vi "view_user_event.vi"(0 "State":string, 5 "Data":variant, 11 "error in (no error)":errorcluster, 13 "Operation":T1) -> (4 "Event Ref":refnum<user-event>, 15 "error out":errorcluster)   [LabVIEW 2020, in "simple_html_chat_ui.lvclass"]
uses:
  simple_html_chat_ui.lvclass
  ui_user_event.ctl
  event_data.ctl
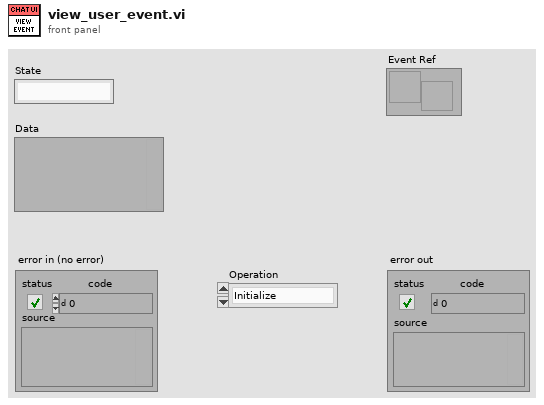
[diagram p1: front panel]
types:
  T1 = typedef "ui_user_event.ctl" = enum16{"Initialize", "Generate", "Get Reference", "Destroy"}
  T2 = typedef "simple_html_chat_ui.lvclass/event_data.ctl" = cluster{"State":string, "Data":variant}
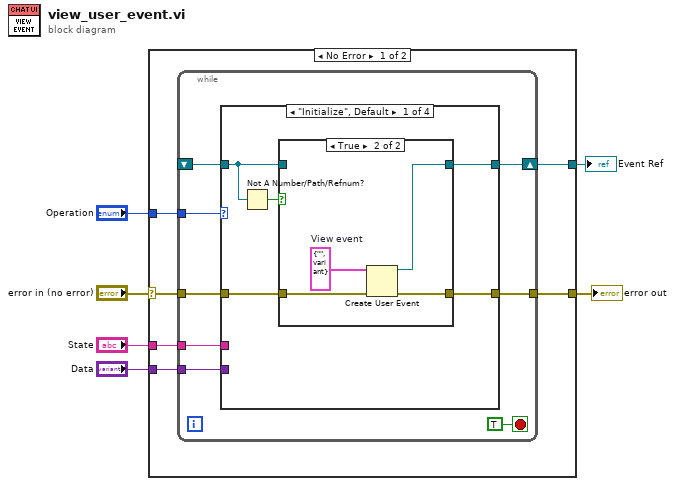
[diagram p0: block diagram]
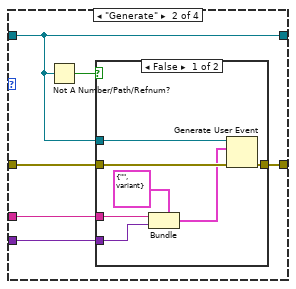
[diagram p3: hidden frame]
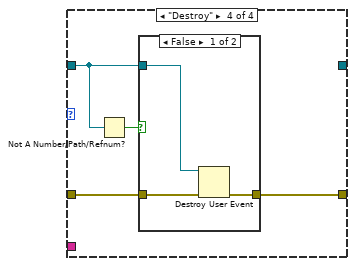
[diagram p6: hidden frame]
diagram:
  n1 = case shown="No Error" "error in (no error)" {
    selector: "error in (no error)" -> [w11 w56]
    tunnel: [w10 w56] -> w5
    tunnel: "Operation" -> [w12 _]
    tunnel: "State" -> [w9 _]
    tunnel: [w8 _] -> w2
    tunnel: "Data" -> [w7 _]
    frame No Error {
      n2 = while {
        tunnel: w12 -> [w19]
        tunnel: w11 -> [w18]
        tunnel: [w17] -> w10
        shift-right: [w16] -> w8
        shift-left: _ -> [w15]
        tunnel: w9 -> [w14]
        tunnel: w7 -> [w13]
        stop <- TRUE stop-if-true
        n3 = case shown="\"Initialize\", Default" w19 {
          tunnel: w18 -> [w25 w37 w46 w51]
          tunnel: [w24 w36 w46 w50] -> w17
          tunnel: [w23 w34 w47 _] -> w16
          tunnel: w15 -> [w21 w34 w47 w48]
          tunnel: w14 -> [_ w33 _ _]
          tunnel: w13 -> [_ w32 _ _]
          frame "Initialize", Default {
            n4 = Not A Number/Path/Refnum?(number/path/refnum=w21) -> (NaN/Path/Refnum?=w22:bool)
            n5 = case shown="True" w22 {
              tunnel: w25 -> [w26 w31]
              tunnel: [w26 w30] -> w24
              tunnel: [w27 w29] -> w23
              tunnel: w21 -> [w27 _]
              frame False {
              }
              frame True {
                w28 = T2 {"State"="", "Data"=variant}  # View event
                n6 = Create User Event(user event datatype=w28, error in=w31) -> (user event=w29:refnum<user-event>, error out=w30:errorcluster)
              }
            }
          }
          frame "Generate" {
            n7 = Not A Number/Path/Refnum?(number/path/refnum=w34) -> (NaN/Path/Refnum?=w35:bool)
            n8 = case shown="False" w35 {
              tunnel: w37 -> [w44 w45]
              tunnel: [w43 w45] -> w36
              tunnel: w34 -> [w42 _]
              tunnel: w33 -> [w40 _]
              tunnel: w32 -> [w39 _]
              frame False {
                n9 = Bundle(cluster=T2 {"State"="", "Data"=variant} ("event data"), "State"=w40, "Data"=w39) -> (w38:T2)
                n10 = Generate User Event(user event=w42, event data cluster=w38, error in=w44) -> (error out=w43:errorcluster)  [unwired: 1 in, 1 out]
              }
              frame True {
              }
            }
          }
          frame "Get Reference" {
          }
          frame "Destroy" {
            n11 = Not A Number/Path/Refnum?(number/path/refnum=w48) -> (NaN/Path/Refnum?=w49:bool)
            n12 = case shown="False" w49 {
              tunnel: w51 -> [w54 w55]
              tunnel: [w53 w55] -> w50
              tunnel: w48 -> [w52 _]
              frame False {
                n13 = Destroy User Event(user event=w52, error in=w54) -> (error out=w53:errorcluster)
              }
              frame True {
              }
            }
          }
        }
      }
    }
    frame Error {
    }
  }
  "error out" <- w5
  "Event Ref" <- w2
